vi "Process.CloseAndStop.vi"(8 "error in":errorcluster, 11 "State Variables":T1) -> (0 "error out":errorcluster, 3 "State Variables":T1)   [LabVIEW 2025, in "xnet_can_bus_monitor_api_server_do.lvlib"]
uses:
  Types/MainProcess.StateVariables.ctl
  Types/XNET.InitialSettings.ctl
  xnet_can_bus_monitor_api_server/RPC Messages/ni_xnet_can_bm_api_ConnectSettings.ctl
  xnet_can_bus_monitor_api_server/RPC Messages/ni_xnet_can_bm_api_CanMode.ctl
  xnet_can_bus_monitor_api_server/RPC Messages/ni_xnet_can_bm_api_Termination.ctl
  xnet_can_bus_monitor_api_server/RPC Messages/ni_xnet_can_bm_api_FdIsoMode.ctl
  xnet_can_bus_monitor_api_server/RPC Messages/ni_xnet_can_bm_api_FilterInfo.ctl
  xnet_can_bus_monitor_api_server/RPC Messages/ni_xnet_can_bm_api_DirectionFilter.ctl
  xnet_can_bus_monitor_api_server/RPC Messages/ni_xnet_can_bm_api_FrameFilter.ctl
  Types/StreamProcess.Refs.ctl
  Types/StreamProcess.VIRef.ctl
  xnet_can_bus_monitor_api_server_do.lvlib
  xnet_can_bus_monitor_api_server/xnet_can_bus_monitor_api_server.lvlib
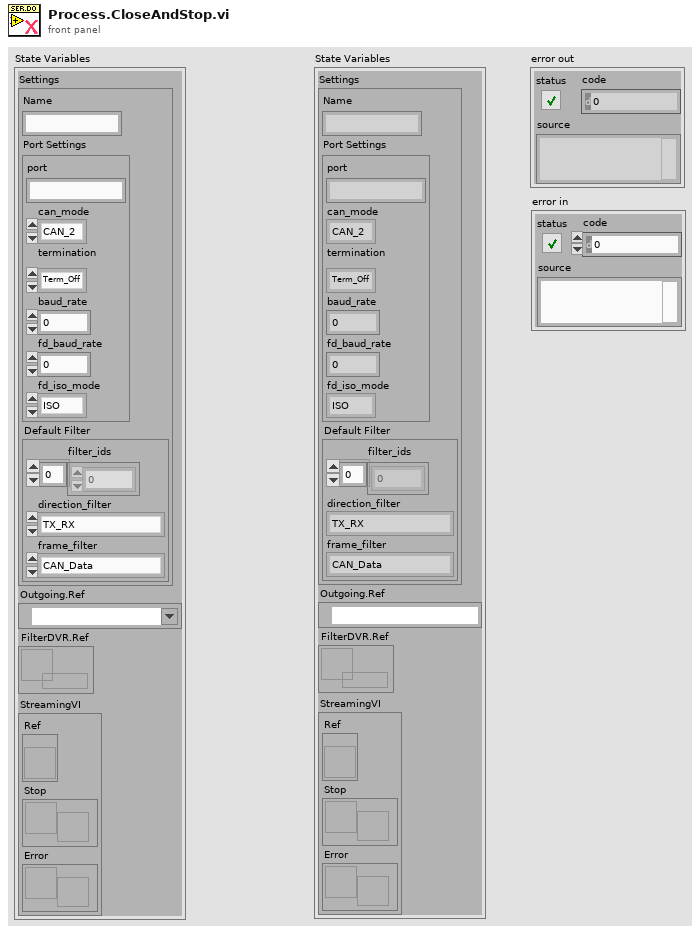
[diagram p1: front panel]
types:
  T1 = typedef "xnet_can_bus_monitor_api_server_do.lvlib/MainProcess.StateVariables.ctl" = cluster{"Settings":T2, "Outgoing.Ref":refnum<k21>, "FilterDVR.Ref":refnum<data-value>, "StreamingVI":T10}
  T2 = typedef "xnet_can_bus_monitor_api_server_do.lvlib/XNET.InitialSettings.ctl" = cluster{"Name":string, "Port Settings":T3, "Default Filter":T7}
  T3 = typedef "xnet_can_bus_monitor_api_server.lvlib/ni_xnet_can_bm_api_ConnectSettings.ctl" = cluster{"port":string, "can_mode":T4, "termination":T5, "baud_rate":u64, "fd_baud_rate":u64, "fd_iso_mode":T6}
  T4 = typedef "xnet_can_bus_monitor_api_server.lvlib/ni_xnet_can_bm_api_CanMode.ctl" = enum32{"CAN_2", "CAN_FD", "CAN_FD_BRS"}
  T5 = typedef "xnet_can_bus_monitor_api_server.lvlib/ni_xnet_can_bm_api_Termination.ctl" = enum32{"Term_Off", "Term_On"}
  T6 = typedef "xnet_can_bus_monitor_api_server.lvlib/ni_xnet_can_bm_api_FdIsoMode.ctl" = enum32{"ISO", "Non_ISO", "ISO_Legacy"}
  T7 = typedef "xnet_can_bus_monitor_api_server.lvlib/ni_xnet_can_bm_api_FilterInfo.ctl" = cluster{"filter_ids":u32[], "direction_filter":T8, "frame_filter":T9}
  T8 = typedef "xnet_can_bus_monitor_api_server.lvlib/ni_xnet_can_bm_api_DirectionFilter.ctl" = enum32{"TX_RX", "RX", "TX"}
  T9 = typedef "xnet_can_bus_monitor_api_server.lvlib/ni_xnet_can_bm_api_FrameFilter.ctl" = enum32{"CAN_Data", "CAN_Remote", "CAN_Bus_Error", "CAN_2_Data", "CAN_FD_Data", "CAN_FD_BRS_Data", "J1939_Data", "Delay", "Log_Trigger", "Start_Trigger", "All"}
  T10 = typedef "xnet_can_bus_monitor_api_server_do.lvlib/StreamProcess.Refs.ctl" = cluster{"Ref":T11, "Stop":refnum<notifier>, "Error":refnum<notifier>}
  T11 = typedef "xnet_can_bus_monitor_api_server_do.lvlib/StreamProcess.VIRef.ctl" = refnum<vi>
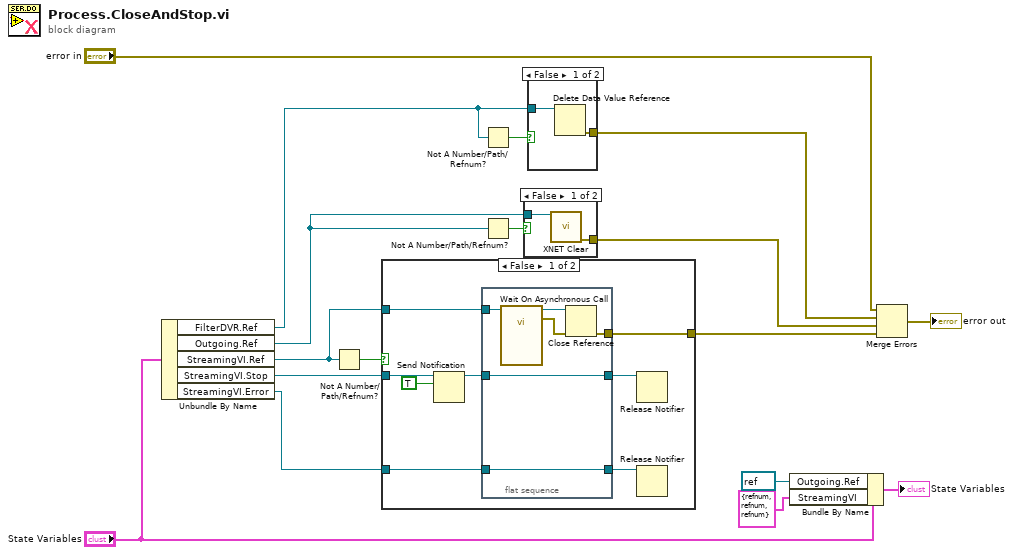
[diagram p0: block diagram]
diagram:
  n1 = Unbundle By Name("State Variables") -> ("FilterDVR.Ref"=w7:refnum<data-value>, "Outgoing.Ref"=w11:refnum<k21>, "StreamingVI.Ref"=w12:T11, "StreamingVI.Stop"=w4:refnum<notifier>, "StreamingVI.Error"=w2:refnum<notifier>)
  n2 = Not A Number/Path/Refnum?(number/path/refnum=w12) -> (NaN/Path/Refnum?=w14:bool)
  n3 = case shown="False" w14 {
    tunnel: w12 -> [w25 _]
    tunnel: [w24 _] -> w16
    tunnel: w4 -> [w22 _]
    tunnel: w2 -> [w18 _]
    frame False {
      n4 = Send Notification(notification=TRUE, notifier=w22) -> (notifier out=w21:refnum<notifier>)  [unwired: 1 in, 1 out]
      n5 = flat-sequence {
        tunnel: w25 -> [w31]
        tunnel: [w28] -> w24
        tunnel: w21 -> [w27]
        tunnel: [w27] -> w20
        tunnel: [w26] -> w19
        tunnel: w18 -> [w26]
        frame #0 {
          n6 = call-by-ref "Wait On Asynchronous Call"(reference=w31) -> (reference out=w30:T11, error out=w29:errorcluster)  [unwired: 12 in, 1 out]
          n7 = Close Reference(reference=w30, error in (no error)=w29) -> (error out=w28:errorcluster)
        }
      }
      n8 = Release Notifier(notifier=w20) -> ()  [unwired: 2 in, 3 out]
      n9 = Release Notifier(notifier=w19) -> ()  [unwired: 2 in, 3 out]
    }
    frame True {
    }
  }
  n10 = Not A Number/Path/Refnum?(number/path/refnum=w7) -> (NaN/Path/Refnum?=w6:bool)
  n11 = Not A Number/Path/Refnum?(number/path/refnum=w11) -> (NaN/Path/Refnum?=w13:bool)
  n12 = case shown="False" w13 {
    tunnel: w11 -> [w33 _]
    tunnel: [w32 _] -> w15
    frame False {
      n13 = call <vilib>:"XNET Clear.vi"("session in"=w33) -> ("error out"=w32:errorcluster)  [unwired: 14 in]
    }
    frame True {
    }
  }
  n14 = case shown="False" w6 {
    tunnel: w7 -> [w35 _]
    tunnel: [w34 _] -> w5
    frame False {
      n15 = Delete Data Value Reference(data value reference=w35) -> (error out=w34:errorcluster)  [unwired: 1 in, 1 out]
    }
    frame True {
    }
  }
  n16 = Bundle By Name(cluster="State Variables", "Outgoing.Ref"=refnum<k21> refnum, "StreamingVI"=T10 {"Ref"=refnum, "Stop"=refnum, "Error"=refnum}) -> (→"State Variables":T1)
  n17 = Merge Errors("error in", w5, w15, w16) -> (→"error out":errorcluster)
